vi "Cryo-Con Get T.vi"(8 "error in (no error)":errorcluster, 10 "Channel":string="A", 11 "VISA Resource Name":refnum<visa-resource-name>) -> (0 "error out":errorcluster, 1 "data string":string, 2 "Temperature":dbl format="%.5f", 3 "VISA Resource Name Out":refnum<visa-resource-name>, 4 "Warning":string)   [LabVIEW 2021]
uses:
  050a9c5d-8ca4-4fe3-8a2a-c323c0318501.vi
  a1aad9ed-9060-41f0-9d69-6282a05df5ca.vi
  <vilib>/Utility/error.llb/Clear Errors.vi
  <vilib>/ErrorRing/Error Ring.xnode
  GPIB/VISA  Send Receive.vi
  Simple VISA Reader/Simple VISA Reader Driver.lvclass
panel:
  out "retries":i32
  out "offset past number":i32
  in  "Array - String":string[](array[string])
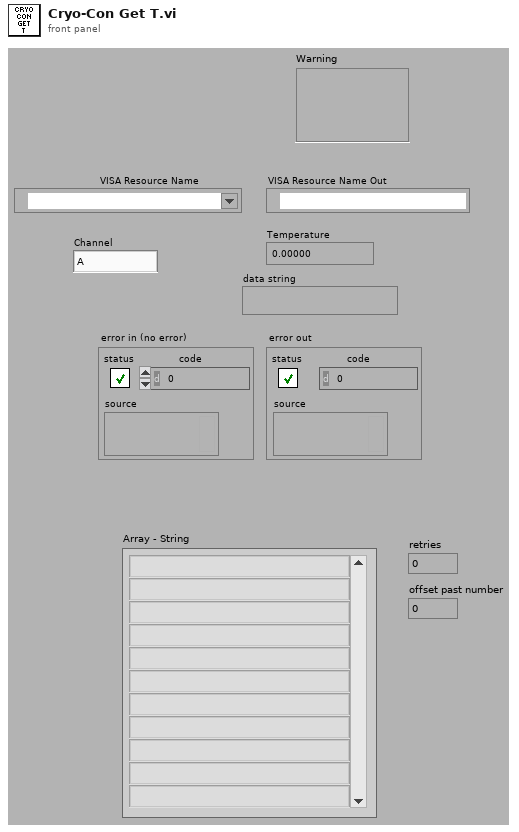
[diagram p1: front panel]
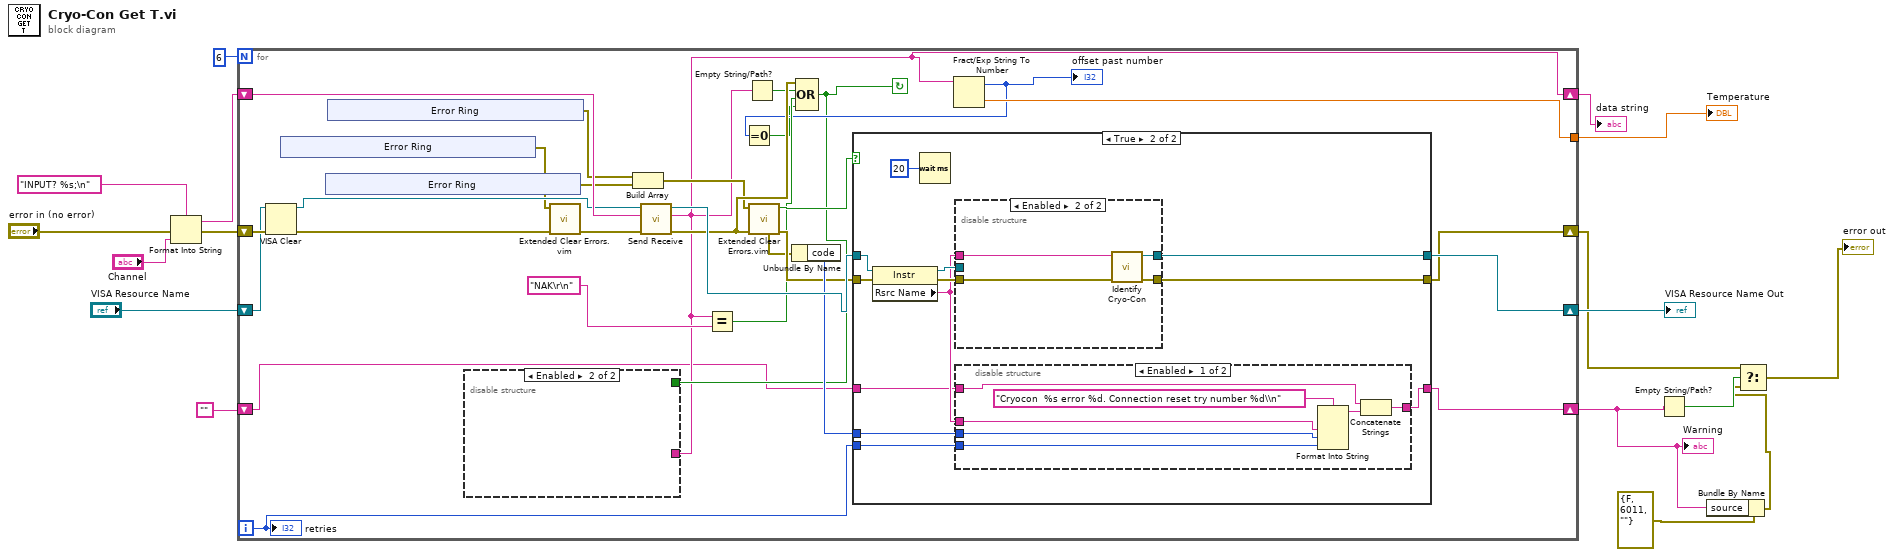
[diagram p0: block diagram]
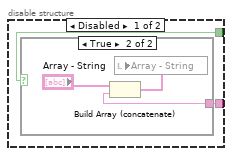
[diagram p2: hidden frame]
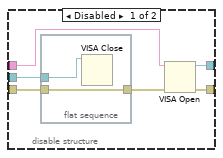
[diagram p5: hidden frame]
diagram:
  n1 = Format Into String(format string="INPUT? %s;\n" ("data string"), error in="error in (no error)", "Channel") -> (resulting string=w12:string, error out=w13:errorcluster)  [unwired: 1 in]
  n2 = for {
    N: 6 -> [_]
    shift-right: [w43] -> w16
    shift-left: "VISA Resource Name" -> [w38]
    shift-right: [w42] -> w5
    shift-left: w13 -> [w40]
    shift-right: [w21] -> w11
    shift-left: w12 -> [w46]
    tunnel: [w25] -> w8
    shift-right: [w19] -> w1
    shift-left: "" -> [w20]
    i -> [w18]
    stop <- w22 continue-if-true
    n3 = VISA Clear(VISA resource name=w38, error in (no error)=w40) -> (VISA resource name out=w39:refnum<visa-resource-name>, error out=w35:errorcluster)
    n4 = xnode "Error Ring"() -> ("error out"=w36:errorcluster)
    n5 = xnode "Error Ring"() -> ("error out"=w37:errorcluster)
    n6 = xnode "Error Ring"() -> ("error out"=w45:errorcluster)
    n7 = call "Extended Clear Errors.vim"("Error In"=w35, "specific error code to clear (0: all)"=w36) -> ("Error Out"=w34:errorcluster)  [unwired: 7 in, 2 out]
    n8 = Build Array(w45, w37) -> (w30:errorcluster[])
    n9 = call-poly "Send Receive.vi"("error in (no error)"=w34, "data string in"=w46, "VISA Resource Name"=w39) -> ("error out"=w33:errorcluster, "data string out"=w21:string, "VISA Resource Name Out"=w44:refnum<visa-resource-name>)  [unwired: 6 in]
    n10 = Equal?(x=w21, y="NAK\r\n") -> (x = y?=w26:bool)
    n11 = Empty String/Path?(string/path=w21) -> (empty?=w28:bool)
    n12 = call "Extended Clear Errors.vim"("Error In"=w33, "specific error code to clear (0: all)"=w30) -> ("Error Out"=w32:errorcluster, "specific error cleared?"=w29:bool, "Original error"=w31:errorcluster)  [unwired: 7 in]
    n13 = Unbundle By Name(w31) -> ("code"=w41:i32)
    n14 = case shown="True" w29 {
      tunnel: w32 -> [w56 w61]
      tunnel: w44 -> [w55 w67]
      tunnel: [w56 w65] -> w42
      tunnel: [w55 w64] -> w43
      tunnel: w41 -> [_ w62]
      tunnel: w20 -> [w54 w57]
      tunnel: [w54 w59] -> w19
      tunnel: w18 -> [_ w58]
      frame False {
      }
      frame True {
        n15 = property class="Instr"(reference=w67, error in=w61) -> (reference out=w68:refnum<visa-resource-name>, error out=w66:errorcluster, "Rsrc Name"=w63:string)
        n16 = Wait (ms)(milliseconds to wait=u32 20) -> ()  [unwired: 1 out]
        n17 = disable-structure shown="Enabled" {
          disable-tunnel: w68 -> [w74 _]
          disable-tunnel: w66 -> [w73 w80]
          disable-tunnel: [w71 w78] -> w65
          disable-tunnel: [w70 w77] -> w64
          disable-tunnel: w63 -> [w69 w79]
          frame Disabled {
            n18 = flat-sequence {
              tunnel: w74 -> [w76]
              tunnel: w73 -> [w75]
              tunnel: [w75] -> w72
              frame #0 {
                n19 = VISA Close(VISA resource name=w76) -> ()  [unwired: 1 in, 1 out]
              }
            }
            n20 = VISA Open(error in (no error)=w72, VISA resource name=w69) -> (VISA resource name=w70:refnum<visa-resource-name>, error out=w71:errorcluster)  [unwired: 3 in]
          }
          frame Enabled {
            n21 = call "Identify Cryo-Con.vi"("Error In"=w80, "VISA resource name"=w79) -> ("Error Out"=w78:errorcluster, "VISA resource name out"=w77:refnum<visa-resource-name>)  [unwired: 6 in, 2 out]
          }
        }
        n22 = disable-structure shown="Enabled" {
          disable-tunnel: w63 -> [w86 _]
          disable-tunnel: w62 -> [w85 _]
          disable-tunnel: [w82 _] -> w59
          disable-tunnel: w58 -> [w83 _]
          disable-tunnel: w57 -> [w81 _]
          frame Enabled {
            n23 = Format Into String(format string="Cryocon  %s error %d. Connection reset try number %d\\n", w86, w85, w83) -> (resulting string=w84:string)  [unwired: 2 in, 1 out]
            n24 = Concatenate Strings(w81, w84) -> (w82:string)
          }
          frame Disabled {
          }
        }
      }
    }
    n25 = Fract/Exp String To Number(string=w21) -> (offset past number=w24:i32, number=w25:dbl)  [unwired: 3 out]
    "offset past number" <- w24
    n26 = Equal To 0?(x=w24) -> (x = 0?=w23:bool)
    n27 = Compound Arithmetic op=OR(w33, w28, w26, w23) -> (w22:bool)
    n28 = disable-structure shown="Enabled" {
      disable-tunnel: w22 -> [w48 _]
      disable-tunnel: w21 -> [w47 _]
      frame Disabled {
        n29 = case shown="True" w48 {
          tunnel: w47 -> [_ w50]
          frame False {
          }
          frame True {
            n30 = Build Array (concatenate)("Array - String", w50) -> (w49:string[])
            n31 = local write "Array - String"(w49) -> ()
          }
        }
      }
      frame Enabled {
      }
    }
    "retries" <- w18
  }
  "data string" <- w11
  "Temperature" <- w8
  "VISA Resource Name Out" <- w16
  "Warning" <- w1
  n32 = Empty String/Path?(string/path=w1) -> (empty?=w6:bool)
  n33 = Bundle By Name(cluster=errorcluster {"status"=FALSE, "code"=6011, "source"=""} ("error constant"), "source"=w1) -> (w2:errorcluster)
  n34 = Select(t=w5, s=w6, f=w2) -> (s? t:f=→"error out":errorcluster)
